vi "Save Submission.vi"(8 "error in (no error)":errorcluster, 10 "Submission":refnum<class "Submission.lvclass">, 11 "Submission DB in":refnum<class "Submission DB.lvclass">) -> (0 "error out":errorcluster, 3 "Submission DB out":refnum<class "Submission DB.lvclass">)   [LabVIEW 2020, in "Summer of LabVIEW.lvlib" / "Submission DB.lvclass"]
uses:
  Submission DB.lvclass
  Submission/Submission.lvclass
  Submission DB.lvclass/Submission DB.ctl
  <vilib>/drjdpowell/SQLite Library/SQL Statement/SQL Statement.lvclass/SQL Statement.ctl
  <vilib>/drjdpowell/SQLite Library/SQL Statement/Bind Text.vi
  <vilib>/drjdpowell/SQLite Library/SQL Statement/Bind Integer.vi
  <vilib>/drjdpowell/SQLite Library/SQL Statement/Step.vi
  <vilib>/drjdpowell/SQLite Library/SQL Statement/Error Message.vi
  SQLite/SQLite.lvclass
  <vilib>/drjdpowell/SQLite Library/SQL Connection/Connection.lvclass
  <vilib>/drjdpowell/SQLite Library/SQL Statement/SQL Statement.lvclass
  <vilib>/IlluminatedG/lv-web-crypto/lv-json/JSON/JSON.lvlib
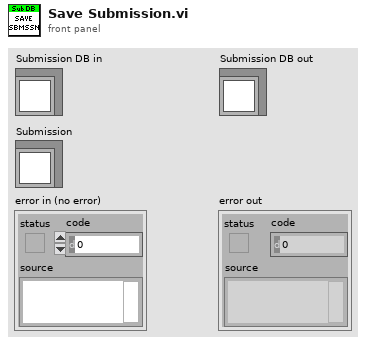
[diagram p1: front panel]
types:
  T1 = typedef "SoL Scoring.lvlib/Score.ctl" = cluster{"Overall":dbl, "Categories":T2[]}
  T2 = typedef "SoL Scoring.lvlib/Score Entry.ctl" = cluster{"Category":string, "Value":dbl}
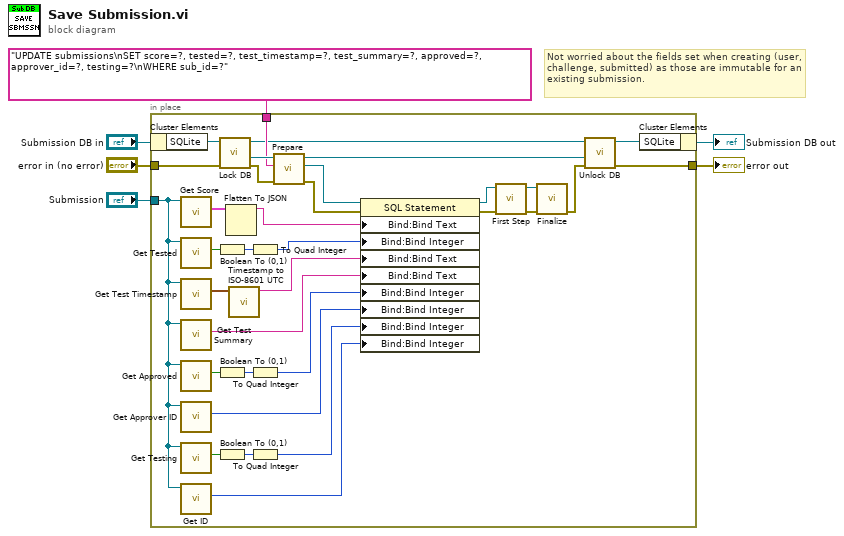
[diagram p0: block diagram]
diagram:
  # "Not worried about the fields set when creating (user, challenge, submitted) as those are immutable for an existing submission."
  n1 = in-place {
    in-place-border: "error in (no error)" -> [w37]
    in-place-border: "UPDATE submissions\nSET score=?, tested=?, test_timestamp=?, test_summary=?, approved=?, approver_id=?, testing=?\nWHERE sub_id=?" ("SQL") -> [w35]
    in-place-border: [w26] -> w3
    in-place-border: "Submission" -> [w11]
    n2 = in-place-cluster #1("Submission DB in") -> ("SQLite"=w38:refnum<class "SQLite.lvclass">)
    n3 = call "Get Score.vi"("Submission in"=w11) -> ("Score"=w23:T1)  [unwired: 9 in, 1 out]
    n4 = call "Get Tested.vi"("Submission in"=w11) -> ("Tested"=w21:bool)  [unwired: 9 in, 1 out]
    n5 = call "Get Test Timestamp.vi"("Submission in"=w11) -> ("Test Timestamp"=w18:timestamp)  [unwired: 9 in, 1 out]
    n6 = call "Get Test Summary.vi"("Submission in"=w11) -> ("Test Summary"=w16:string)  [unwired: 9 in, 1 out]
    n7 = call "Get Approved.vi"("Submission in"=w11) -> ("Approved"=w14:bool)  [unwired: 9 in, 1 out]
    n8 = call "Get Approver ID.vi"("Submission in"=w11) -> ("Approver ID"=w12:i64)  [unwired: 9 in, 1 out]
    n9 = call "Get Testing.vi"("Submission in"=w11) -> ("Testing"=w9:bool)  [unwired: 9 in, 1 out]
    n10 = call "Get ID.vi"("Submission in"=w11) -> ("ID"=w7:i64)  [unwired: 9 in, 1 out]
    n11 = Boolean To (0,1)(Boolean=w21) -> (0, 1=w20:i16)
    n12 = Boolean To (0,1)(Boolean=w14) -> (0, 1=w15:i16)
    n13 = Boolean To (0,1)(Boolean=w9) -> (0, 1=w10:i16)
    n14 = call "Lock DB.vi"("error in (no error)"=w37, "SQLite in"=w38) -> ("error out"=w39:errorcluster, "SQLite DB"=w36:refnum<class "Connection.lvclass">, "SQLite out"=w28:refnum<class "SQLite.lvclass">)  [unwired: 6 in, 1 out]
    n15 = Flatten To JSON(anything=w23) -> (JSON string=w22:string)  [unwired: 2 in, 1 out]
    n16 = call <vilib>:"Timestamp to ISO-8601 UTC.vi"("Time Stamp"=w18) -> ("ISO 8601 UTC"=w17:string)  [unwired: 10 in]
    n17 = To Quad Integer(1:w20) -> (0:w19:i64)
    n18 = To Quad Integer(1:w15) -> (0:w13:i64)
    n19 = To Quad Integer(1:w10) -> (0:w8:i64)
    n20 = call <vilib>:"Prepare.vi"("error in (no error)"=w39, "SQL"=w35, "SQLite Connection in"=w36) -> ("error out"=w33:errorcluster, "SQL Statement"=w34:refnum<class "SQL Statement.lvclass">, "SQLite Connection"=w24:refnum<class "Connection.lvclass">)  [unwired: 4 in, 2 out]
    n21 = property class="SQL Statement"(reference=w34, error in=w33, "Bind:Bind Text"=w22, "Bind:Bind Integer"=w19, "Bind:Bind Text"=w17, "Bind:Bind Text"=w16, "Bind:Bind Integer"=w13, "Bind:Bind Integer"=w12, "Bind:Bind Integer"=w8, "Bind:Bind Integer"=w7) -> (reference out=w30:refnum<class "SQL Statement.lvclass">, error out=w32:errorcluster)
    n22 = call <vilib>:"First Step.vi"("error in (no error)"=w32, "SQL Statement in"=w30) -> ("error out"=w31:errorcluster, "SQL Statement"=w29:refnum<class "SQL Statement.lvclass">)  [unwired: 7 in, 1 out]
    n23 = call <vilib>:"Finalize.vi"("error in (no error)"=w31, "SQL Statement in"=w29) -> ("error out"=w25:errorcluster)  [unwired: 9 in]
    n24 = call "Unlock DB.vi"("error in (no error)"=w25, "SQLite DB"=w24, "SQLite in"=w28) -> ("error out"=w26:errorcluster, "SQLite out"=w27:refnum<class "SQLite.lvclass">)  [unwired: 7 in]
    n25 = in-place-cluster #1("SQLite"=w27) -> (→"Submission DB out":refnum<class "Submission DB.lvclass">)
  }
  "error out" <- w3
